vi "Remove form.vi"(8 "error in (no error)":errorcluster, 10 "Form ID":T1, 11 "Update Fields Logic Simple Table in":refnum<class "Update Fields Logic Simple Table.lvclass">) -> (0 "error out":errorcluster, 3 "Update Fields Logic Simple Table out":refnum<class "Update Fields Logic Simple Table.lvclass">)   [LabVIEW 2020, in "Update Fields Logic Simple Table.lvlib" / "Update Fields Logic Simple Table.lvclass"]
uses:
  Update Fields Logic Simple Table.lvclass
  Autoclose manager/Form ID.ctl
  Update Fields Logic Simple Table.lvclass/Update Fields Logic Simple Table.ctl
  <userlib>/_OpenG.lib/array/array.llb/Search 1D Array (Variant)__ogtk.vi
  <userlib>/_OpenG.lib/array/array.llb/Delete Elements from 1D Array (String)__ogtk.vi
  <userlib>/_OpenG.lib/array/array.llb/Delete Elements from 1D Array (Variant)__ogtk.vi
  Form Server Interfaces.lvlib
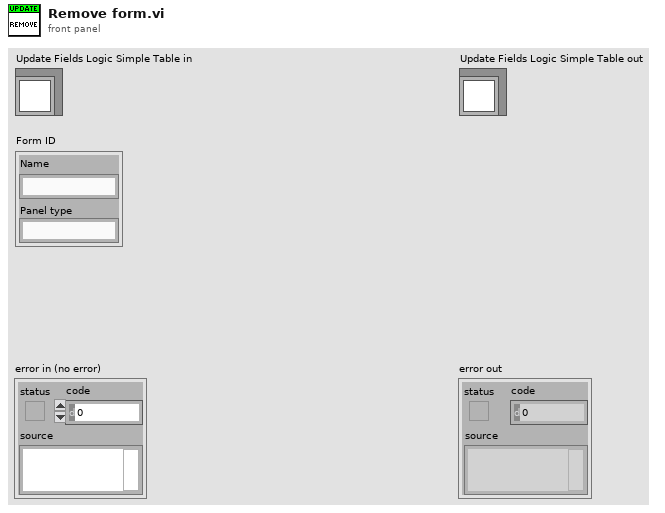
[diagram p1: front panel]
types:
  T1 = typedef "Form Server Interfaces.lvlib/Form ID.ctl" = cluster{"Name":string, "Panel type":string}
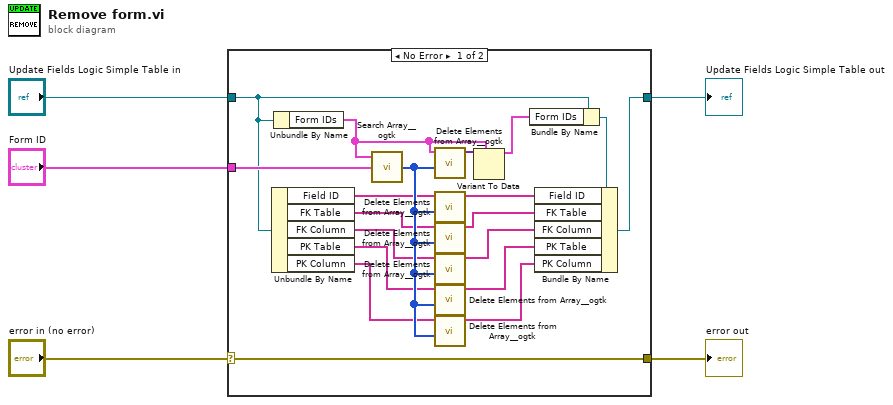
[diagram p0: block diagram]
diagram:
  n1 = case shown="No Error" "error in (no error)" {
    selector: "error in (no error)" -> [w24 w26]
    tunnel: [w24 w26] -> w1
    tunnel: "Update Fields Logic Simple Table in" -> [w14 w25]
    tunnel: [w12 w25] -> w3
    tunnel: "Form ID" -> [w23 _]
    frame No Error {
      n2 = Unbundle By Name(w14) -> ("Field ID"=w15:string[], "FK Table"=w21:string[], "FK Column"=w20:string[], "PK Table"=w19:string[], "PK Column"=w18:string[])
      n3 = Unbundle By Name(w14) -> ("Form IDs"=w16:T1[])
      n4 = call-poly <userlib>:"Search Array__ogtk.vi"("Array"=w16, "Element Data"=w23) -> ("Indices of Elements"=w22:i32[])  [unwired: 7 in]
      n5 = call-poly <userlib>:"Delete Elements from Array__ogtk.vi"("indices"=w22, "array"=w16) -> ("array w/ subset deleted"=w17:variant[])  [unwired: 8 in, 1 out]
      n6 = call-poly <userlib>:"Delete Elements from Array__ogtk.vi"("indices"=w22, "array"=w15) -> ("array w/ subset deleted"=w10:string[])  [unwired: 8 in, 1 out]
      n7 = call-poly <userlib>:"Delete Elements from Array__ogtk.vi"("indices"=w22, "array"=w21) -> ("array w/ subset deleted"=w9:string[])  [unwired: 8 in, 1 out]
      n8 = call-poly <userlib>:"Delete Elements from Array__ogtk.vi"("indices"=w22, "array"=w20) -> ("array w/ subset deleted"=w8:string[])  [unwired: 8 in, 1 out]
      n9 = call-poly <userlib>:"Delete Elements from Array__ogtk.vi"("indices"=w22, "array"=w19) -> ("array w/ subset deleted"=w7:string[])  [unwired: 8 in, 1 out]
      n10 = call-poly <userlib>:"Delete Elements from Array__ogtk.vi"("indices"=w22, "array"=w18) -> ("array w/ subset deleted"=w6:string[])  [unwired: 8 in, 1 out]
      n11 = Variant To Data(type=w16, Variant=w17) -> (data=w11:T1[])  [unwired: 1 in, 1 out]
      n12 = Bundle By Name(cluster=w14, "Form IDs"=w11) -> (w13:refnum<class "Update Fields Logic Simple Table.lvclass">)
      n13 = Bundle By Name(cluster=w13, "Field ID"=w10, "FK Table"=w9, "FK Column"=w8, "PK Table"=w7, "PK Column"=w6) -> (w12:refnum<class "Update Fields Logic Simple Table.lvclass">)
    }
    frame Error {
    }
  }
  "error out" <- w1
  "Update Fields Logic Simple Table out" <- w3
